vi "thscan_comparator_mpix.vi"() -> ()   [LabVIEW 2022 SP3]
panel:
  in  "Tab Control":enum32{"Single", "ROI"}(tab)
  out "ThScan_SP":u16[][](graph)
  out "ThScans_ROI":u16[][](graph)
  in  "Current File":u16(ring)=1 items=["RED", "BLUE"]
  in  "file blue":path=path "C:/Users/User/OneDrive/measurements/mpix/2023-04-14_pommiary_RK_testowe_przed_RG/0050mA/7a_ikrum=  2; igm= 32; vt0=  s; vt1=   ; DIS_DYN_SW= ; MPR_en= ; bgshc_W= ; bgshc_N= ; bgshc_NW= ;/0.bin"
  in  "file red":path=path "C:/Users/User/OneDrive/measurements/mpix/2023-04-14_pommiary_RK_testowe_przed_RG/0100mA/7a_ikrum=  2; igm= 32; vt0=  s; vt1=   ; DIS_DYN_SW= ; MPR_en= ; bgshc_W= ; bgshc_N= ; bgshc_NW= ;/0.bin"
  out "MainImg":u16[][](graph)
  in  "ThScan_Load":bool
  in  "Exit":bool
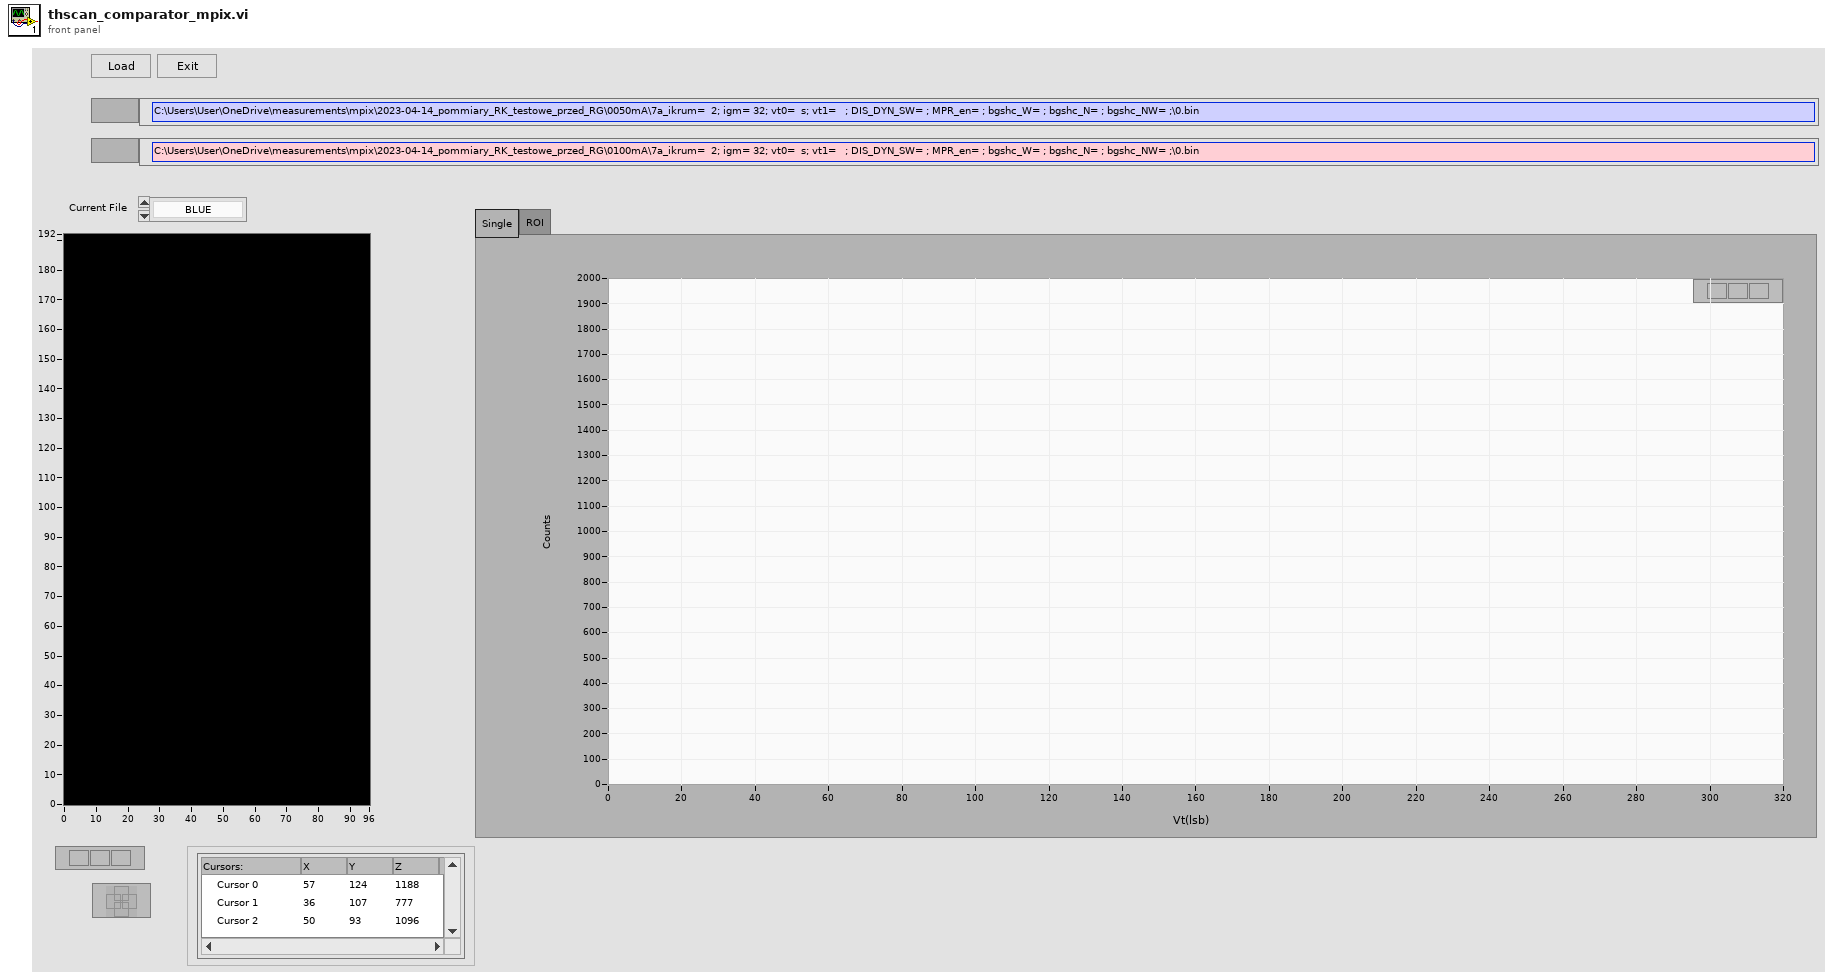
[diagram p1: front panel]
types:
  T1 = enum16{"big-endian, network order", "native, host order", "little-endian"}
  T2 = typedef "LVPointDoubleTypeDef.ctl" = cluster{"Cursor X":dbl, "Cursor Y":dbl}
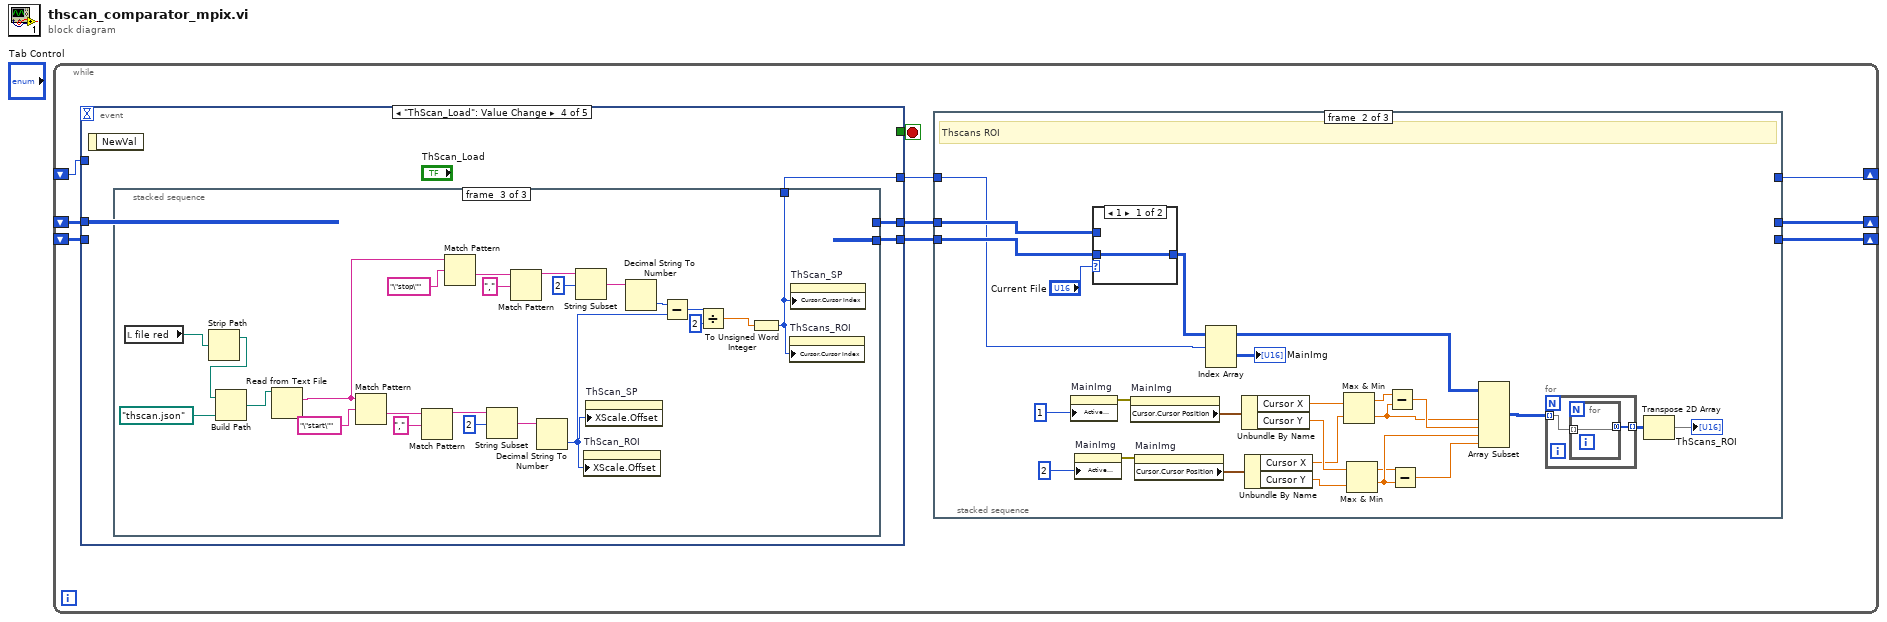
[diagram p0: block diagram]
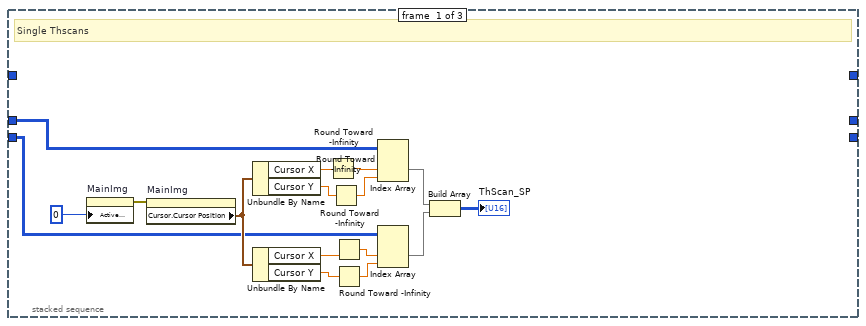
[diagram p2: hidden frame]
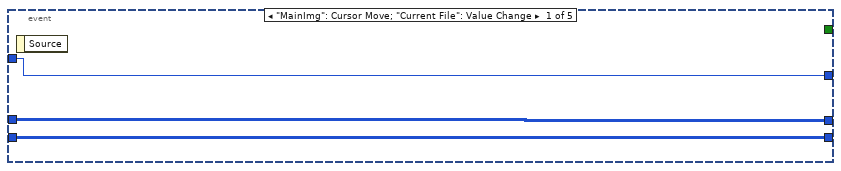
[diagram p5: hidden frame]
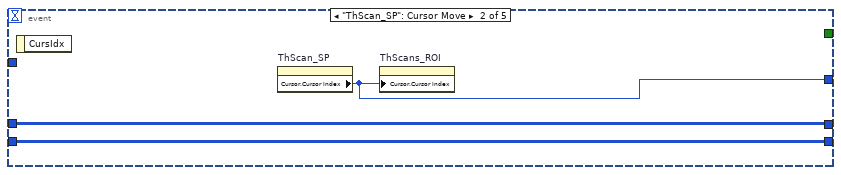
[diagram p6: hidden frame]
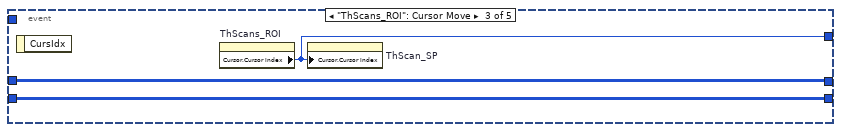
[diagram p7: hidden frame]
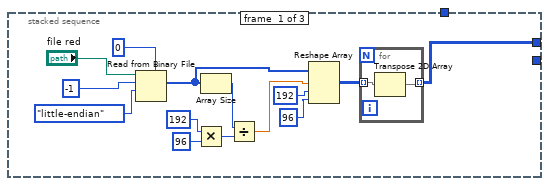
[diagram p8: hidden frame]
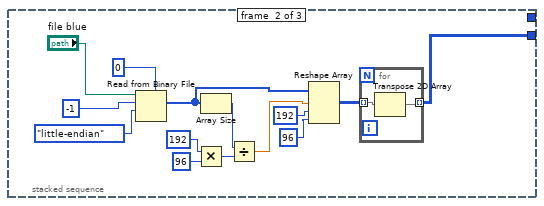
[diagram p9: hidden frame]
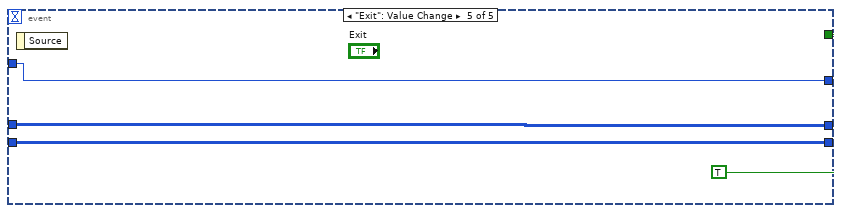
[diagram p10: hidden frame]
diagram:
  n1 = while {
    shift-right: [w4] -> _
    shift-left: _ -> [w9]
    shift-right: [w5] -> _
    shift-left: _ -> [w8]
    shift-right: [w2] -> _
    shift-left: _ -> [w1]
    stop <- w10 stop-if-true
    n2 = event shown="[3] \"ThScan_Load\": Value Change" {
      selector: _ -> [_ _ _ _ _]
      dyn-events: _ -> [_ _ _ _ _]
      timeout: _ -> [_ _ _ _ _]
      tunnel: [_ _ _ _ TRUE] -> w10
      tunnel: w9 -> [w62 w64 w67 _ w129]
      tunnel: [w62 w64 w67 w71 w129] -> w7
      tunnel: [w61 w65 w68 w70 w128] -> w6
      tunnel: w8 -> [w61 w65 w68 _ w128]
      tunnel: [w60 w63 w66 w69 w127] -> w3
      tunnel: w1 -> [w60 _ _ _ w127]
      event "MainImg": Cursor Move; "Current File": Value Change {
        n3 = event-data() -> ()  [unwired: 1 in, 1 out]
      }
      event "ThScan_SP": Cursor Move {
        n4 = event-data() -> ()  [unwired: 1 in, 1 out]
        n5 = property on="ThScan_SP" class="WFGraph (strict)"() -> ("Cursor.Cursor Index"=w63:i32)  [unwired: 2 in, 2 out]
        n6 = property on="ThScans_ROI" class="WFGraph (strict)"("Cursor.Cursor Index"=w63) -> ()  [unwired: 2 in, 2 out]
      }
      event "ThScans_ROI": Cursor Move {
        n7 = event-data() -> ()  [unwired: 1 in, 1 out]
        n8 = property on="ThScans_ROI" class="WFGraph (strict)"() -> ("Cursor.Cursor Index"=w66:i32)  [unwired: 2 in, 2 out]
        n9 = property on="ThScan_SP" class="WFGraph (strict)"("Cursor.Cursor Index"=w66) -> ()  [unwired: 2 in, 2 out]
      }
      event "ThScan_Load": Value Change {
        n10 = event-data() -> ()  [unwired: 1 in, 1 out]
        n11 = stacked-sequence {
          tunnel: [_ w88 _] -> w71
          tunnel: [w73 _ _] -> w70
          tunnel: [_ _ w104] -> w69
          frame #0 {
            n12 = Read from Binary File(5:u16 0, 9:T1."little-endian" ("byte order (0:big-endian, network order)"), 10:-1 ("count (1)"), 11:"file red") -> (2:w84:u16[])  [unwired: 2 in, 3 out]
            n13 = Multiply(x=192 ("dimension size"), y=96 ("dimension size")) -> (x*y=w82:i32)
            n14 = Array Size(array=w84) -> (size(s)=w81:i32)
            n15 = Divide(x=w81, y=w82) -> (x/y=w83:dbl)
            n16 = Reshape Array(w84, w83, 192 ("dimension size"), 96 ("dimension size")) -> (w85:u16[][][])
            n17 = for {
              tunnel: w85 -> [w87] mode=indexing
              tunnel: [w86] -> w73 mode=indexing
              n18 = Transpose 2D Array(2D array=w87) -> (transposed array=w86:u16[][])
            }
          }
          frame #1 {
            n19 = Read from Binary File(5:u16 0, 9:T1."little-endian" ("byte order (0:big-endian, network order)"), 10:-1 ("count (1)"), 11:"file blue") -> (2:w98:u16[])  [unwired: 2 in, 3 out]
            n20 = Multiply(x=192 ("dimension size"), y=96 ("dimension size")) -> (x*y=w100:i32)
            n21 = Array Size(array=w98) -> (size(s)=w101:i32)
            n22 = Divide(x=w101, y=w100) -> (x/y=w99:dbl)
            n23 = Reshape Array(w98, w99, 192 ("dimension size"), 96 ("dimension size")) -> (w97:u16[][][])
            n24 = for {
              tunnel: w97 -> [w103] mode=indexing
              tunnel: [w102] -> w88 mode=indexing
              n25 = Transpose 2D Array(2D array=w103) -> (transposed array=w102:u16[][])
            }
          }
          frame #2 {
            n26 = local read "file red"() -> (w106:path)
            n27 = Strip Path(path=w106) -> (stripped path=w105:path)  [unwired: 1 out]
            n28 = Build Path(base path=w105, name or relative path=path "thscan.json") -> (appended path=w123:path)
            n29 = Read from Text File(file (use dialog)=w123) -> (text=w112:string)  [unwired: 3 in, 3 out]
            n30 = Match Pattern(string=w112, regular expression="\"start\"") -> (after substring=w124:string)  [unwired: 1 in, 3 out]
            n31 = Match Pattern(string=w124, regular expression=",") -> (before substring=w125:string)  [unwired: 1 in, 3 out]
            n32 = Match Pattern(string=w112, regular expression="\"stop\"") -> (after substring=w116:string)  [unwired: 1 in, 3 out]
            n33 = String Subset(string=w125, offset (0)=2) -> (substring=w126:string)  [unwired: 1 in]
            n34 = Match Pattern(string=w116, regular expression=",") -> (before substring=w117:string)  [unwired: 1 in, 3 out]
            n35 = Decimal String To Number(string=w126) -> (number=w108:i32)  [unwired: 2 in, 1 out]
            n36 = String Subset(string=w117, offset (0)=2) -> (substring=w118:string)  [unwired: 1 in]
            n37 = property on="ThScan_ROI" class="WFGraph (strict)"("XScale.Offset"=w108) -> ()  [unwired: 2 in, 2 out]
            n38 = property on="ThScan_SP" class="WFGraph (strict)"("XScale.Offset"=w108) -> ()  [unwired: 2 in, 2 out]
            n39 = Decimal String To Number(string=w118) -> (number=w111:i32)  [unwired: 2 in, 1 out]
            n40 = Subtract(x=w111, y=w108) -> (x-y=w110:i32)
            n41 = Divide(x=w110, y=2) -> (x/y=w107:dbl)
            n42 = To Unsigned Word Integer(number=w107) -> (unsigned 16bit integer=w104:u16)
            n43 = property on="ThScans_ROI" class="WFGraph (strict)"("Cursor.Cursor Index"=w104) -> ()  [unwired: 2 in, 2 out]
            n44 = property on="ThScan_SP" class="WFGraph (strict)"("Cursor.Cursor Index"=w104) -> ()  [unwired: 2 in, 2 out]
          }
        }
      }
      event "Exit": Value Change {
        n45 = event-data() -> ()  [unwired: 1 in, 1 out]
      }
    }
    n46 = stacked-sequence {
      tunnel: w7 -> [w11 w28 w58]
      tunnel: w6 -> [w12 w29 w59]
      tunnel: [_ _ w59] -> w5
      tunnel: [_ _ w58] -> w4
      tunnel: w3 -> [_ w27 w57]
      tunnel: [_ _ w57] -> w2
      frame #0 {
        # "Single Thscans"
        n47 = property on="MainImg" class="IntGraph (strict)"("Active Cursor"=u32 0) -> (error out=w14:errorcluster)  [unwired: 2 in, 1 out]
        n48 = property on="MainImg" class="IntGraph (strict)"(error in=w14) -> ("Cursor.Cursor Position"=w15:T2)  [unwired: 1 in, 2 out]
        n49 = Unbundle By Name(w15) -> ("Cursor X"=w24:dbl, "Cursor Y"=w25:dbl)
        n50 = Unbundle By Name(w15) -> ("Cursor X"=w20:dbl, "Cursor Y"=w21:dbl)
        n51 = Round Toward -Infinity(1:w24) -> (0:w23:dbl)
        n52 = Round Toward -Infinity(1:w25) -> (0:w26:dbl)
        n53 = Round Toward -Infinity(1:w20) -> (0:w19:dbl)
        n54 = Round Toward -Infinity(1:w21) -> (0:w22:dbl)
        n55 = Index Array(array=w12, index (dim 1)=w23, index (dim 2)=w26) -> (element=w18:u16[])  [unwired: 1 in]
        n56 = Index Array(array=w11, index (dim 1)=w19, index (dim 2)=w22) -> (element=w17:u16[])  [unwired: 1 in]
        n57 = Build Array(w18, w17) -> (→"ThScan_SP":u16[][])
      }
      frame #1 {
        # "Thscans ROI"
        n58 = property on="MainImg" class="IntGraph (strict)"("Active Cursor"=u32 1) -> (error out=w36:errorcluster)  [unwired: 2 in, 1 out]
        n59 = property on="MainImg" class="IntGraph (strict)"("Active Cursor"=u32 2) -> (error out=w37:errorcluster)  [unwired: 2 in, 1 out]
        n60 = case shown="1" "Current File" {
          tunnel: w29 -> [_ w56]
          tunnel: w28 -> [w55 _]
          tunnel: [w55 w56] -> w50
          frame 1 {
          }
          frame 0, Default {
          }
        }
        n61 = property on="MainImg" class="IntGraph (strict)"(error in=w36) -> ("Cursor.Cursor Position"=w38:T2)  [unwired: 1 in, 2 out]
        n62 = property on="MainImg" class="IntGraph (strict)"(error in=w37) -> ("Cursor.Cursor Position"=w39:T2)  [unwired: 1 in, 2 out]
        n63 = Index Array(array=w50, index (dim 0)=w27) -> (element=→"MainImg":u16[][])  [unwired: 2 in]
        n64 = Unbundle By Name(w38) -> ("Cursor X"=w40:dbl, "Cursor Y"=w42:dbl)
        n65 = Unbundle By Name(w39) -> ("Cursor X"=w41:dbl, "Cursor Y"=w43:dbl)
        n66 = Max & Min(x=w40, y=w41) -> (max(x,y)=w44:dbl, min(x,y)=w45:dbl)
        n67 = Max & Min(x=w42, y=w43) -> (max(x,y)=w47:dbl, min(x,y)=w49:dbl)
        n68 = Subtract(x=w44, y=w45) -> (x-y=w46:dbl)
        n69 = Subtract(x=w47, y=w49) -> (x-y=w48:dbl)
        n70 = Array Subset(array=w50, index (dim 1)=w45, length (dim 1)=w46, index (dim 2)=w49, length (dim 2)=w48) -> (w34:u16[][][])  [unwired: 2 in]
        n71 = for {
          tunnel: [w53] -> w33 mode=indexing
          tunnel: w34 -> [w52] mode=indexing
          n72 = for {
            tunnel: w52 -> [w54] mode=indexing
            tunnel: [w54] -> w53 mode=concatenating
          }
        }
        n73 = Transpose 2D Array(2D array=w33) -> (transposed array=→"ThScans_ROI":u16[][])
      }
      frame #2 {
      }
    }
  }
